vi "TDC_writeTimestamps.vi"(8 "Error In":errorcluster, 10 "Data Format":i32(ring) items=["Ascii", "Binary", "Compressed", "Raw", "None"], 11 "Path":path) -> (0 "Error Out":errorcluster)   [LabVIEW 2011]
uses:
  tdcbase.dll
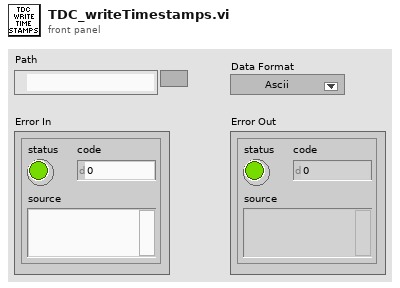
[diagram p1: front panel]
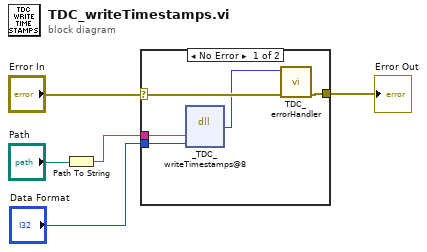
[diagram p0: block diagram]
diagram:
  n1 = Path To String(path="Path") -> (string=w2:string)
  n2 = case shown="No Error" "Error In" {
    selector: "Error In" -> [w9 w11]
    tunnel: [w8 w11] -> w4
    tunnel: w2 -> [w10 _]
    tunnel: "Data Format" -> [w6 _]
    frame No Error {
      n3 = dll-call lib="X:/tdcbase.dll" fn="_TDC_writeTimestamps@8"("filename"=w10, "format"=w6) -> ("return type"=w7:i32)  [unwired: 5 in, 2 out]
      n4 = call "TDC_errorHandler.vi"("Error In"=w9, "TDC Return Code"=w7) -> ("Error Out"=w8:errorcluster)  [unwired: 9 in]
    }
    frame Error {
    }
  }
  "Error Out" <- w4
